vi "AlliGator Fit Linear Combinations of Exponentials.vi"(0 "Fit Simulation Parameters":T13, 5 "Decay Simulation Parameters":T14, 7 "Decay Fit Options & Parameters":T2 {"Fit Options"."Offset Resolution" min=0.0; "Fit Options"."Period" min=0.0; "Fit Options"."Min Decay Percentile" min=0.0 max=1.0; "Fit Options"."Max Decay Percentile" min=0.0 max=100.0; "Fit Parameter Constraints"."Max Value" format="%#.3g"; "Fit Parameter Constraints"."Min Value" format="%#.3g"}, 9 "Reference Decay":cluster{"t Array":dbl[], "IRF Array":dbl[]}, 11 "Error In":errorcluster, 12 "Show Decays, Fits & Residuals":bool) -> (1 "Output Plots":cluster{"t Array":dbl[], "I Array":dbl[]}[](array[cluster]), 2 "Output Plot Names":string[](array[string]), 3 "Plot Colors":u32[](array[colorbox]), 4 "Fit Results":T1[](array[typedef]), 6 "tau 1":dbl[](array[numeric]), 8 "tau 2":dbl[](array[numeric]), 10 "a 1":dbl[](array[numeric]), 14 "Message":string, 15 "Error Out":errorcluster)   [LabVIEW 2021, in "AlliGator Fit Method Benchmark.lvlib"]
doc: "Simulate a 1-Exp or 2-Exp decay and fits it with the selected model."
uses:
  AlliGator Fit Method Benchmark.lvlib
  AlliGator Decay Simulation Parameters.ctl
  AlliGator Fit Simulation Parameters.ctl
  AlliGator Decay Fit Options & Parameters v2.ctl
  Fits/IRF(X)PSED/Decay Fit Options v2.ctl
  Fits/Decay Convolution/Decay Model.ctl
  Fits/Residual Type.ctl
  Fits/IRF(X)PSED/Fit Weights Type.ctl
  Fits/Non-linear Fitting Method v2.ctl
  Fits/Fit Calculation Method.ctl
  Fits/Non-linear Fitting Algorithm.ctl
  AlliGator Decay Fit Parameter Constraints 2.ctl
  Fits/IRF(X)PSED/Decay Fit Parameters In List.ctl
  Fits/IRF(X)PSED/MLE Baseline Offset Type.ctl
  Fits/IRF(X)PSED/IRF(X)PSED Fit Results.ctl
  Histograms/Linear Histogram Options.ctl
  Histograms/Histogram Bin Option.ctl
  Histograms/Histogram Bin Position.ctl
  Graphs/XY Graph/XY Graph Selected Plot Info+Flag.ctl
  Graphs/XY Graph/XY Graph Refnum.ctl
  <vilib>/Utility/miscctls.llb/LVPoint32TypeDef.ctl
  593261b4-01b2-4f61-a03e-748a91d26851.vi
  593261b4-01b2-4f61-a03e-748a91d26851.vi/e021cd17-e000-4244-b7f4-ec50548bdfcb.vi
  593261b4-01b2-4f61-a03e-748a91d26851.vi/b1828c6e-eb0a-43e9-a724-8b596c52e435.vi
  593261b4-01b2-4f61-a03e-748a91d26851.vi/7a6138ed-c001-4311-b538-9ba42ae7c7b1.vi
  593261b4-01b2-4f61-a03e-748a91d26851.vi/52c6b4fa-501b-4af0-803b-8bab516ca5d3.vi
  593261b4-01b2-4f61-a03e-748a91d26851.vi/d7237e10-35ab-4bcb-a0c6-4883c3f4c990.vi
  593261b4-01b2-4f61-a03e-748a91d26851.vi/5fb5dd96-3b97-4592-ba56-58181c8e7105.vi
  593261b4-01b2-4f61-a03e-748a91d26851.vi/8e13a849-a393-4484-9968-4af7b25c38d7.vi
  <vilib>/Utility/error.llb/Error Cluster From Error Code.vi
  AlliGator Abort.vi
  <vilib>/gmath/statdist.llb/Uniform (Discrete) Random.vi
  <userlib>/_OpenG.lib/array/array.llb/Filter 1D Array__ogtk.vi
  <userlib>/_OpenG.lib/array/array.llb/Filter 1D Array (DBL)__ogtk.vi
  <userlib>/_OpenG.lib/array/array.llb/Delete Elements from Array__ogtk.vi
  <userlib>/_OpenG.lib/array/array.llb/Delete Elements from 1D Array (DBL)__ogtk.vi
  <vilib>/ErrorRing/Error Ring.xnode
  Histograms/Histogram Window.lvlib
  Math/Math.lvlib
  GUI/GUI.lvlib
  AlliGator Globals, Variables & Constants.lvlib
  Time/Time.lvlib
  Variant/Variant.lvlib
  AlliGator Decay Fit.lvlib
  Graphs/XY Graph/XY Graph Add-Ons.lvlib
  Fits/Fits.lvlib
  <vilib>/gmath/NI_Gmath.lvlib
  Error/Error.lvlib
  <vilib>/gmath/statdist.llb/Exp Random.vi
  AlliGator Decay Fit Parameter Map.lvlib
panel:
  # "see the AlliGator License on the block diagram (Ctrl+E or Window:Show Block Diagram)"
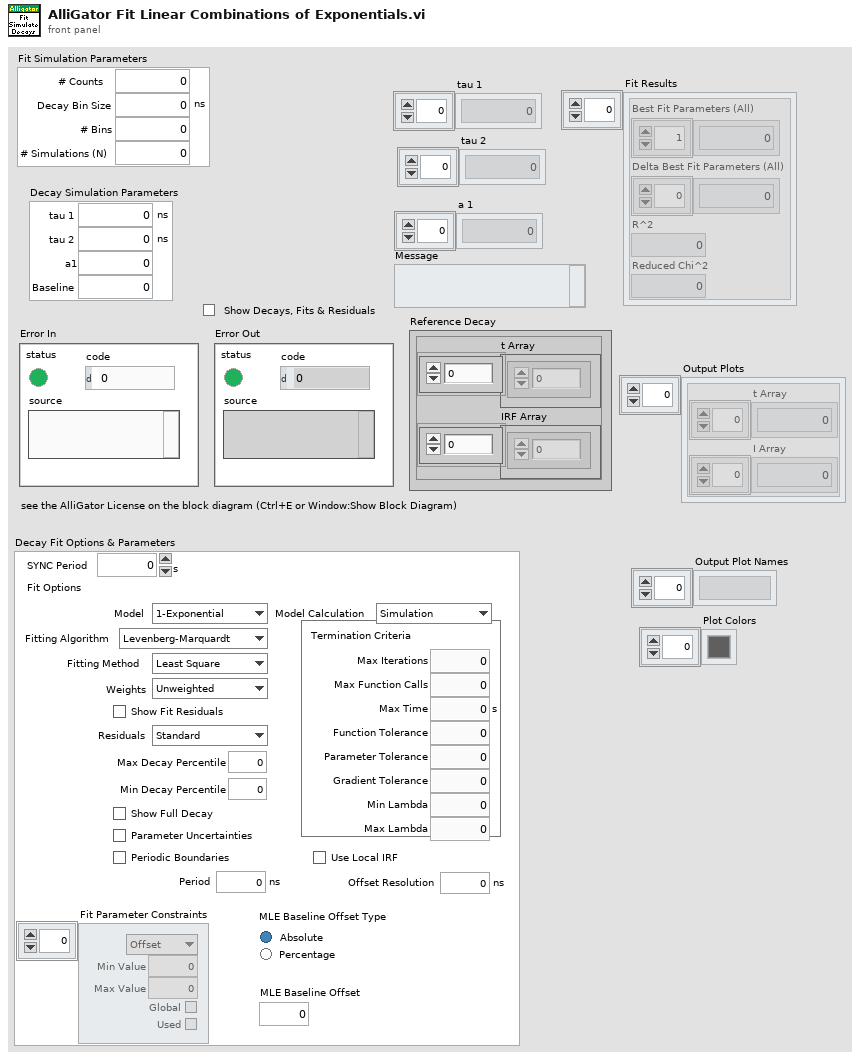
[diagram p1: front panel]
types:
  T1 = typedef "Fits.lvlib/IRF(X)PSED Fit Results.ctl" = cluster{"Best Fit Parameters (All)":dbl[], "Delta Best Fit Parameters (All)":dbl[], "R^2":dbl, "Reduced Chi^2":dbl}
  T2 = typedef "AlliGator Decay Fit Parameter Map.lvlib/AlliGator Decay Fit Options & Parameters v2.ctl" = cluster{"SYNC Period":dbl[unit], "Fit Options":T3, "Fit Parameter Constraints":T10[], "MLE Baseline Offset":dbl, "MLE Baseline Offset Type":T12}
  T3 = typedef "Fits.lvlib/Decay Fit Options v2.ctl" = cluster{"Show Fit Residuals":bool, "Fit Model":T4, "Residual Type":T5, "Max Decay Percentile":dbl, "Min Decay Percentile":dbl, "Show Full Decay":bool, "Weights":T6, "Fitting Method":T7, "Compute Parameter Uncertainties":bool, "Periodic Boundaries":bool, "Model Calculation":T8, "Period":dbl[unit], "Termination Criteria":cluster{"Max Iterations":i32, "Max Function Calls":i32, "Max Time":dbl[unit], "Function Tolerance":dbl, "Parameter Tolerance":dbl, "Gradient Tolerance":dbl, "Min Lambda":dbl, "Max Lambda":dbl, "Initial Tick Count":u32}, "Offset Resolution":dbl[unit], "Use Local IRF":bool, "Fitting Algorithm":T9}
  T4 = typedef "Fits.lvlib/Decay Model.ctl" = enum16{"1-Exponential", "2-Exponentials"}
  T5 = typedef "Fits.lvlib/Residual Type.ctl" = enum16{"Standard", "Normalized", "Reduced"}
  T6 = typedef "Fits.lvlib/Fit Weights Type.ctl" = enum16{"Unweighted", "1/Variance", "Best of All"}
  T7 = typedef "Fits.lvlib/Non-linear Fitting Method v2.ctl" = enum16{"Least Square", "Least Absolute Residual", "Bisquare", "MLE", "-", "Best of All"}
  T8 = typedef "Fits.lvlib/Fit Calculation Method.ctl" = enum16{"Simulation", "Convolution", "Integration"}
  T9 = typedef "Fits.lvlib/Non-linear Fitting Algorithm.ctl" = enum16{"Levenberg-Marquardt", "Trust-Region Dogleg"}
  T10 = typedef "AlliGator Decay Analysis.lvlib/AlliGator Decay Fit.lvlib/AlliGator Decay Fit Parameter Constraints 2.ctl" = cluster{"Fit Parameter":T11, "Min Value":dbl, "Max Value":dbl, "Global":bool, "Used":bool}
  T11 = typedef "Fits.lvlib/Decay Fit Parameters In List.ctl" = enum16{"Offset", "Baseline", "A_1", "tau_1", "A_2", "tau_2"}
  T12 = typedef "Fits.lvlib/MLE Baseline Offset Type.ctl" = enum32{"Absolute", "Percentage"}
  T13 = typedef "AlliGator Fit Method Benchmark.lvlib/AlliGator Fit Simulation Parameters.ctl" = cluster{"# Counts":i32, "# Simulations (N)":i32, "Decay Bin Size":dbl[unit], "# Bins":i32}
  T14 = typedef "AlliGator Fit Method Benchmark.lvlib/AlliGator Decay Simulation Parameters.ctl" = cluster{"tau 1":dbl[unit], "tau 2":dbl[unit], "a1":dbl, "Baseline":dbl}
  T15 = typedef "Histogram Window.lvlib/Linear Histogram Options.ctl" = cluster{"Bin Size":dbl, "Bin Number":i32, "Bin Option":T16, "Min Value":dbl, "Max Value":dbl, "Filter NaN & Infinite Values":bool, "Frequency Plot":bool, "Align Bins":bool, "Bin Location":T17, "Project Outside Values":bool, "Max Histogram Size":i32}
  T16 = typedef "Histogram Window.lvlib/Histogram Bin Option.ctl" = enum32{"Bin Number", "Bin Size"}
  T17 = typedef "Histogram Window.lvlib/Histogram Bin Position.ctl" = enum16{"Left", "Center", "Right"}
  T18 = typedef "XY Graph Add-Ons.lvlib/XY Graph Selected Plot Info+Flag.ctl" = cluster{"Multiplot XY Graph":T19, "Mouse Coordinates":T20, "Plot Index":i32, "Flag":bool}
  T19 = typedef "XY Graph Add-Ons.lvlib/XY Graph Refnum.ctl" = refnum<vi>
  T20 = typedef "LVPoint32TypeDef.ctl" = cluster{"Horizontal":i32, "Vertical":i32}
  T21 = typedef "XY Graph Add-Ons.lvlib/XY Plot Data.ctl" = cluster{"X Array":dbl[], "Y Array":dbl[]}
  T22 = cluster{"t Array":dbl[], "Intensity Array":dbl[]}[]
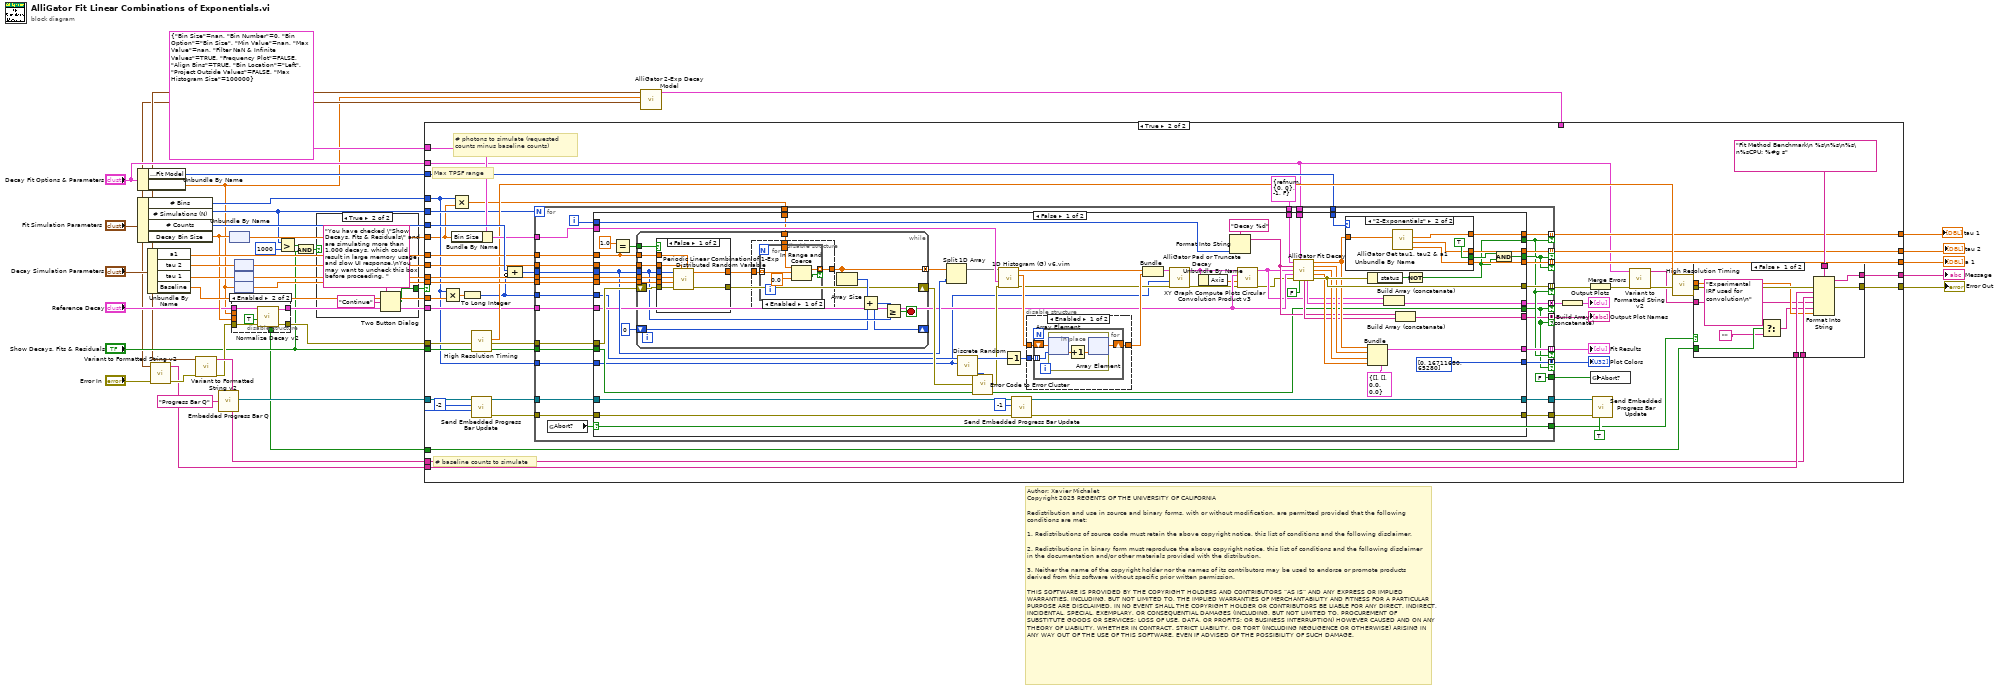
[diagram p0: block diagram]
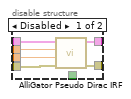
[diagram p2: hidden frame]
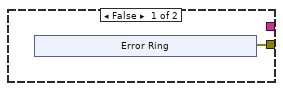
[diagram p3: hidden frame]
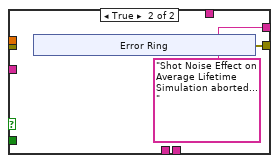
[diagram p4: hidden frame]
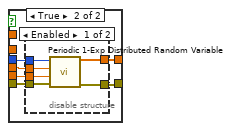
[diagram p6: hidden frame]
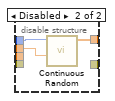
[diagram p7: hidden frame]
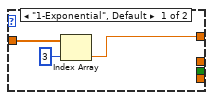
[diagram p9: hidden frame]
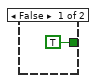
[diagram p11: hidden frame]
diagram:
  # "Author: Xavier Michalet\nCopyright 2025 REGENTS OF THE UNIVERSITY OF CALIFORNIA\n\nRedistribution and use in source and binary forms, with or without modification, are permitted provided that the following conditions are met:\n\n1. Redistributions of source code must retain the above copyright notice, this list of conditions and the following disclaimer.\n\n2. Redistributions in binary form must reproduce the above copyright notice, this list of conditions and the following disclaimer in the documentation and/or other materials provided with the distribution.\n\n3. Neither the name of the copyright holder nor the names of its contributors may be used to endorse or promote products derived from this software without specific prior written permission.\n\nTHIS SOFTWARE IS PROVIDED BY THE COPYRIGHT HOLDERS AND CONTRIBUTORS “AS IS” AND ANY EXPRESS OR IMPLIED WARRANTIES, INCLUDING, BUT NOT LIMITED TO, THE IMPLIED WARRANTIES OF MERCHANTABILITY AND FITNESS FOR A PARTICULAR PURPOSE ARE DISCLAIMED. IN NO EVENT SHALL THE COPYRIGHT HOLDER OR CONTRIBUTORS BE LIABLE FOR ANY DIRECT, INDIRECT, INCIDENTAL, SPECIAL, EXEMPLARY, OR CONSEQUENTIAL DAMAGES (INCLUDING, BUT NOT LIMITED TO, PROCUREMENT OF SUBSTITUTE GOODS OR SERVICES; LOSS OF USE, DATA, OR PROFITS; OR BUSINESS INTERRUPTION) HOWEVER CAUSED AND ON ANY THEORY OF LIABILITY, WHETHER IN CONTRACT, STRICT LIABILITY, OR TORT (INCLUDING NEGLIGENCE OR OTHERWISE) ARISING IN ANY WAY OUT OF THE USE OF THIS SOFTWARE, EVEN IF ADVISED OF THE POSSIBILITY OF SUCH DAMAGE."
  n1 = Unbundle By Name("Decay Fit Options & Parameters") -> ("Fit Options.Fit Model"=w23:T4, "Fit Options.Period"=w2:dbl[unit])
  n2 = Unbundle By Name("Fit Simulation Parameters") -> ("# Bins"=w6:i32, "# Simulations (N)"=w13:i32, "# Counts"=w40:i32, "Decay Bin Size"=w17:dbl[unit])
  n3 = Unbundle By Name("Decay Simulation Parameters") -> ("a1"=w37:dbl, "tau 2"=w35:dbl[unit], "tau 1"=w36:dbl[unit], "Baseline"=w19:dbl)
  n4 = call "Variant to Formatted String v2.vi"("error in (no error)"="Error In", "Anything"="Fit Simulation Parameters") -> ("error out"=w26:errorcluster, "String"=w25:string)  [unwired: 8 in]
  n5 = call "Variant to Formatted String v2.vi"("error in (no error)"=w26, "Anything"="Decay Simulation Parameters") -> ("error out"=w15:errorcluster, "String"=w24:string)  [unwired: 8 in]
  n6 = call "Embedded Progress Bar Q.vi"("Progress Bar Queue Name"="Progress Bar Q") -> ("Progress Bar Queue"=w30:refnum<queue>)  [unwired: 6 in]
  n7 = node(w17) -> (w32:dbl)
  n8 = disable-structure shown="Enabled" {
    disable-tunnel: [w46 w50] -> w18
    disable-tunnel: w17 -> [w45 _]
    disable-tunnel: "Reference Decay" -> [w44 w52]
    disable-tunnel: w15 -> [w43 w51]
    disable-tunnel: [w42 w49] -> w14
    disable-tunnel: w2 -> [w41 _]
    disable-tunnel: [_ w47] -> w5
    frame Disabled {
      n9 = call "AlliGator Pseudo Dirac IRF.vi"("Error In"=w43, "Decay Bin Size"=w45, "Period"=w41, "Reference Decay in"=w44) -> ("Error Out"=w42:errorcluster, "Reference Decay out"=w46:cluster{"t Array":dbl[], "IRF Array":dbl[]})  [unwired: 6 in]
    }
    frame Enabled {
      n10 = call "Normalize Decay v2.vi"("Error In"=w51, "Max = 1 (F)/Integral = 1 (T)"=TRUE, "Decay"=w52) -> ("Error Out"=w49:errorcluster, "Normalized Decay"=w50:cluster{"t Array":dbl[], "Y Array":dbl[]}, "Is Valid Plot?"=w47:bool)  [unwired: 4 in, 2 out]
    }
  }
  n11 = node(w35) -> (w33:dbl)
  n12 = node(w36) -> (w34:dbl)
  n13 = node(w2) -> (w39:dbl)
  n14 = Greater?(x=w13, y=1000) -> (0:w11:bool)
  n15 = And(x=w11, y="Show Decays, Fits & Residuals") -> (x .and. y?=w9:bool)
  n16 = case shown="True" w9 {
    tunnel: [TRUE ("T button?") w54] -> w8
    frame False {
    }
    frame True {
      n17 = Two Button Dialog(message="You have checked \"Show Decays, Fits & Residuals\" and are simulating more than 1,000 decays, which could result in large memory usage and slow UI response.\nYou may want to uncheck this box before proceeding. ", 2:"Continue" ("T button name (\"OK\")")) -> (T button?=w54:bool)  [unwired: 1 in]
    }
  }
  n18 = call "AlliGator 2-Exp Decay Model.vi"("Fit Simulation Parameters"="Fit Simulation Parameters", "Period"=w2, "Decay Simulation Parameters"="Decay Simulation Parameters") -> ("Output Plot"=w1:cluster{"t Array":dbl[], "I Array":dbl[]})  [unwired: 8 in]
  n19 = case shown="True" w8 {
    tunnel: w40 -> [_ w113]
    tunnel: w39 -> [_ w112]
    tunnel: T15 {"Bin Size"=nan, "Bin Number"=0, "Bin Option"=enum."Bin Size", "Min Value"=nan, "Max Value"=nan, "Filter NaN & Infinite Values"=TRUE, "Frequency Plot"=FALSE, "Align Bins"=TRUE, "Bin Location"=enum."Left", "Project Outside Values"=FALSE, "Max Histogram Size"=100000} ("Histogram Options") -> [_ w111]
    tunnel: w37 -> [_ w109]
    tunnel: w34 -> [_ w108]
    tunnel: w33 -> [_ w107]
    tunnel: w32 -> [_ w65]
    tunnel: w30 -> [_ w105]
    tunnel: [w57 w98] -> w29
    tunnel: [_ w97] -> w28
    tunnel: w25 -> [_ w96]
    tunnel: w24 -> [_ w95]
    tunnel: w23 -> [_ w86]
    tunnel: [_ w85] -> w22
    tunnel: [_ w84] -> w21
    tunnel: [_ w83] -> w20
    tunnel: "Decay Fit Options & Parameters" -> [_ w80]
    tunnel: w19 -> [_ w70]
    tunnel: w18 -> [_ w74]
    tunnel: w14 -> [_ w73]
    tunnel: w13 -> [_ w72]
    tunnel: "Show Decays, Fits & Residuals" -> [_ w71]
    tunnel: w6 -> [_ w66]
    tunnel: w5 -> [_ w63]
    tunnel: w1 -> [_ _]
    frame False {
      n20 = xnode "Error Ring"() -> ("error out"=w57:errorcluster)
    }
    frame True {
      # "Max TPSF range"
      # "# photons to simulate (requested counts minus baseline counts)"
      # "# baseline counts to simulate"
      n21 = Multiply(x=w66, y=w70) -> (x*y=w69:dbl)
      n22 = Multiply(x=w66, y=w65) -> (x*y=w64:dbl)
      n23 = Bundle By Name(cluster=w111, "Bin Size"=w65) -> (w110:T15)
      n24 = To Long Integer(number=w69) -> (32bit integer=w67:i32)
      n25 = call "High Resolution Timing.vi"("Error In"=w73) -> ("elapsed (relative) seconds"=w91:dbl, "Error Out"=w93:errorcluster)  [unwired: 16 in, 1 out]
      n26 = call "Send Embedded Progress Bar Update.vi"("Max Iterations N"=w72, "Current Iteration i (i or -1: standard or || iteration; 0 or -2: first standard or || iteration)"=-2 ("Current Iteration i (-1: || iteration, -2: first || iteration)"), "Progress Bar Queue in"=w105) -> ("Error Out"=w102:errorcluster, "Progress Bar Queue out"=w104:refnum<queue>)  [unwired: 7 in]
      n27 = Compound Arithmetic op=ADD(w113, invert w67) -> (w68:i32)
      n28 = for {
        N: w72 -> [_]
        tunnel: w68 -> [w164]
        tunnel: w112 -> [w163]
        tunnel: w93 -> [w162]
        tunnel: w110 -> [w161]
        tunnel: w109 -> [w145]
        tunnel: w108 -> [w160]
        tunnel: w107 -> [w159]
        tunnel: w102 -> [w156]
        tunnel: [w155] -> w101
        tunnel: [FALSE ("Abort?")] -> w99
        tunnel: [w142] -> w89
        tunnel: w74 -> [w153]
        tunnel: w80 -> [w151]
        tunnel: [w144] -> w88 mode=indexing if=w140
        tunnel: T18 {"Multiplot XY Graph"=refnum, "Mouse Coordinates"={"Horizontal"=0, "Vertical"=0}, "Plot Index"=-1, "Flag"=FALSE} ("Selected Plot Info + Flag") -> [w150]
        tunnel: w86 -> [w149]
        tunnel: [w148] -> w85 mode=indexing if=w140
        tunnel: [w147] -> w84 mode=indexing if=w141
        tunnel: [w146] -> w83 mode=indexing if=w141
        tunnel: w104 -> [w158]
        tunnel: [w157] -> w103
        tunnel: [w143] -> w78 mode=indexing if=w140
        tunnel: [w139] -> w76 mode=concatenating if=w132
        tunnel: [w138] -> w77 mode=concatenating if=w132
        tunnel: w71 -> [w137]
        tunnel: [w136] -> w75 mode=concatenating if=w132
        tunnel: w67 -> [w135]
        tunnel: w66 -> [w134]
        tunnel: w64 -> [w133]
        i -> [w152]
        n29 = global read "AlliGator Abort.vi" "Abort?"() -> (w142:bool)
        n30 = case shown="False" w142 {
          tunnel: w164 -> [w177 _]
          tunnel: w163 -> [w227 _]
          tunnel: w162 -> [w226 w294]
          tunnel: w161 -> [w225 _]
          tunnel: w160 -> [w224 _]
          tunnel: w159 -> [w223 _]
          tunnel: w158 -> [w221 w293]
          tunnel: [w220 w293] -> w157
          tunnel: w156 -> [w219 w292]
          tunnel: [w218 w292] -> w155
          tunnel: w153 -> [w175 _]
          tunnel: w152 -> [w217 _]
          tunnel: w151 -> [w215 _]
          tunnel: w150 -> [w213 _]
          tunnel: w149 -> [w212 _]
          tunnel: [w211 _] -> w148
          tunnel: [w210 _] -> w147
          tunnel: [w208 _] -> w146
          tunnel: w145 -> [w207 _]
          tunnel: [w204 w294] -> w144
          tunnel: [w202 _] -> w141
          tunnel: [w201 _] -> w140
          tunnel: [w195 _] -> w143
          tunnel: [w190 _] -> w139
          tunnel: [w191 _] -> w138
          tunnel: [w183 _] -> w132
          tunnel: w137 -> [w183 _]
          tunnel: [u32[] [0, 16711680, 65280] ("Plot Colors (Default)") _] -> w136
          tunnel: w135 -> [w170 _]
          tunnel: w134 -> [w167 _]
          tunnel: w133 -> [w184 _]
          frame False {
            n31 = Equal?(x=1.0, y=w207) -> (x = y?=w206:bool)
            n32 = while {
              tunnel: w227 -> [w242]
              tunnel: w224 -> [w240]
              tunnel: w223 -> [w239]
              tunnel: w207 -> [w238]
              tunnel: w206 -> [w237]
              tunnel: w184 -> [w235]
              tunnel: [w234] -> w182 mode=concatenating
              tunnel: w177 -> [w233]
              shift-right: [w228] -> w179
              shift-left: w226 -> [w241]
              shift-right: [w229] -> _
              shift-left: 0 -> [w230]
              stop <- w232 stop-if-true
              n33 = case shown="False" w237 {
                tunnel: w233 -> [w259 w263]
                tunnel: w242 -> [w258 w261]
                tunnel: w241 -> [w257 w265]
                tunnel: [w256 w260] -> w236
                tunnel: [w255 w264] -> w228
                tunnel: w240 -> [w254 w262]
                tunnel: w239 -> [w253 _]
                tunnel: w238 -> [w252 _]
                frame False {
                  n34 = call "Periodic Linear Combination of 1-Exp Distributed Random Variable.vi"("a 1 (in [0, 1])"=w252, "tau 2"=w253, "Error In"=w257, "T"=w258, "tau 1"=w254, "# Elements"=w259) -> ("Error Out"=w255:errorcluster, "t Array"=w256:dbl[])  [unwired: 4 in]
                }
                frame True {
                  n35 = disable-structure shown="Enabled" {
                    disable-tunnel: w265 -> [w271 _]
                    disable-tunnel: [w270 _] -> w264
                    disable-tunnel: w263 -> [w269 w274]
                    disable-tunnel: w262 -> [w268 w273]
                    disable-tunnel: w261 -> [w267 _]
                    disable-tunnel: [w266 w272] -> w260
                    frame Enabled {
                      n36 = call "Periodic 1-Exp Distributed Random Variable.vi"("Error In"=w271, "T"=w267, "tau"=w268, "# Elements"=w269) -> ("Error Out"=w270:errorcluster, "t Array"=w266:dbl[])  [unwired: 6 in]
                    }
                    frame Disabled {
                      n37 = call-poly <vilib>:"Continuous Random.vi"("b"=w273, "samples"=w274) -> ("exp random data"=w272:dbl[])  [unwired: 8 in, 1 out]
                    }
                  }
                }
              }
              n38 = disable-structure shown="Enabled" {
                disable-tunnel: w236 -> [w245 w251]
                disable-tunnel: w235 -> [w244 _]
                disable-tunnel: [w243 w251] -> w234
                frame Enabled {
                  n39 = for {
                    tunnel: w245 -> [w249] mode=indexing
                    tunnel: w244 -> [w250]
                    tunnel: [w247] -> w243 mode=indexing if=w246
                    n40 = In Range and Coerce(upper limit=w250, x=w249, lower limit=0.0 ("x")) -> (coerced(x)=w247:dbl, In Range?=w246:bool)
                  }
                }
                frame Disabled {
                }
              }
              n41 = Array Size(array=w234) -> (size(s)=w231:i32)
              n42 = Add(x=w231, y=w230) -> (x+y=w229:i32)
              n43 = Greater Or Equal?(x=w229, y=w233) -> (x >= y?=w232:bool)
            }
            n44 = Split 1D Array(array=w182, index=w177) -> (first subarray=w176:dbl[])  [unwired: 1 out]
            n45 = call-poly <vilib>:"Discrete Random.vi"("n"=w167, "samples"=w170) -> ("error"=w180:i32, "uniform (discrete) random data"=w188:i32[])  [unwired: 8 in]
            n46 = call "Error Code to Error Cluster.vi"("Error Code"=w180, "Error In"=w179) -> ("Error Out"=w178:errorcluster)  [unwired: 13 in]
            n47 = call "1D Histogram (G) v6.vim"("Error In"=w178, "Histogram Options"=w225, "Array"=w176) -> ("Error Out"=w169:errorcluster, "Histogram"=w186:dbl[], "Axis"=w171:dbl[])  [unwired: 2 in, 4 out]
            n48 = Decrement(x=w188) -> (x-1=w187:i32[])
            n49 = call "Send Embedded Progress Bar Update.vi"("Error In"=w219, "Current Iteration i (i or -1: standard or || iteration; 0 or -2: first standard or || iteration)"=-1 ("Current Iteration i (i or -1: standard or || iteration; 0 or -2: first standard or || iteration)"), "Progress Bar Queue in"=w221) -> ("Error Out"=w218:errorcluster, "Progress Bar Queue out"=w220:refnum<queue>)  [unwired: 7 in]
            n50 = disable-structure shown="Enabled" {
              disable-tunnel: w187 -> [w277 _]
              disable-tunnel: w186 -> [w276 w283]
              disable-tunnel: [w275 w283] -> w185
              frame Enabled {
                n51 = for {
                  tunnel: w277 -> [w278] mode=indexing
                  shift-right: [w279] -> w275
                  shift-left: w276 -> [w280]
                  n52 = in-place {
                    n53 = in-place-array #1(w280, w278) -> (w282:dbl)
                    n54 = Increment(x=w282) -> (x+1=w281:dbl)
                    n55 = in-place-array #1(w281) -> (w279:dbl[])  [unwired: 1 out]
                  }
                }
              }
              frame Disabled {
              }
            }
            n56 = Bundle("Axis"=w171, "Histogram"=w185) -> (w172:cluster{"Axis":dbl[], "Histogram":dbl[]})  [unwired: 1 in]
            n57 = call "AlliGator Pad or Truncate Decay.vi"("Error In"=w169, "# Requested Points"=w167, "Plot in"=w172) -> ("Error Out"=w168:errorcluster, "Plot out"=w166:cluster{"Axis":dbl[], "Histogram":dbl[]})  [unwired: 7 in]
            n58 = Unbundle By Name(w166) -> ("Axis"=w165:dbl[])
            n59 = Format Into String(format string="Decay %d", w217) -> (resulting string=w189:string)  [unwired: 2 in, 1 out]
            n60 = call "XY Graph Compute Plots Circular Convolution Product v3.vi"("Error In"=w168, "Support Axis (kernel's)"=w165, "Plot 2 (kernel)"=w175, "Plot 1 (function)"=w166) -> ("Error Out"=w173:errorcluster, "Convolution Product"=w174:T21)  [unwired: 5 in, 1 out]
            n61 = call "AlliGator Fit Decay.vi"("Selected Plot Info + Flag"=w213, "Decay Fit Options & Parameters"=w215, "Current Decay Name"=w189, "Current Decay"=w174, "Reference Decay"=w175, "error in (no error)"=w173, "Use Legacy Fitting Approach"=FALSE) -> ("Output Plots"=w193:T22, "Best Fit Parameters (All)"=w200:dbl[], "Delta Best Fit Parameters (All)"=w199:dbl[], "R^2"=w198:dbl, "Reduced Chi^2"=w197:dbl, "Output Plot Names"=w194:string[], "Error Out"=w204:errorcluster)  [unwired: 2 out]
            n62 = case shown="\"2-Exponentials\"" w212 {
              tunnel: w200 -> [w286 w290]
              tunnel: [w284 w289] -> w211
              tunnel: [_ w288] -> w210
              tunnel: [_ TRUE] -> w209
              tunnel: [_ w287] -> w208
              frame "1-Exponential", Default {
                n63 = Index Array(array=w286, index=3) -> (element=w284:dbl)
              }
              frame "2-Exponentials" {
                n64 = call "AlliGator Get tau1, tau2 & a1.vi"("Best Fit Parameters"=w290) -> ("a 1"=w287:dbl, "tau 2"=w288:dbl, "tau 1"=w289:dbl)  [unwired: 8 in]
              }
            }
            n65 = Unbundle By Name(w204) -> ("status"=w203:bool)
            n66 = Bundle(cluster=T1 {"Best Fit Parameters (All)"=[], "Delta Best Fit Parameters (All)"=[], "R^2"=0.0, "Reduced Chi^2"=0.0} ("output cluster"), "Best Fit Parameters (All)"=w200, "Delta Best Fit Parameters (All)"=w199, "R^2"=w198, "Reduced Chi^2"=w197) -> (w195:T1)
            n67 = Build Array (concatenate)(w174, w193) -> (w191:T21[])
            n68 = Build Array (concatenate)(w189, w194) -> (w190:string[])
            n69 = Not(x=w203) -> (.not. x?=w201:bool)
            n70 = And(x=w209, y=w201) -> (x .and. y?=w202:bool)
          }
          frame True {
          }
        }
      }
      "Fit Results" <- w78
      "Output Plot Names" <- w76
      "Plot Colors" <- w75
      n71 = Build Array (concatenate)(w77) -> (→"Output Plots":T21[])
      n72 = Merge Errors(w88) -> (w82:errorcluster)
      n73 = global write "AlliGator Abort.vi" "Abort?"(w99) -> ()
      n74 = call "Send Embedded Progress Bar Update.vi"("Stop Progress Bar (F)"=TRUE, "Error In"=w101, "Progress Bar Queue in"=w103) -> ()  [unwired: 7 in, 2 out]
      n75 = call "Variant to Formatted String v2.vi"("error in (no error)"=w82, "Anything"=w80) -> ("error out"=w81:errorcluster, "String"=w79:string)  [unwired: 8 in]
      n76 = call "High Resolution Timing.vi"("relative seconds (NaN)"=w91, "Error In"=w81) -> ("elapsed (relative) seconds"=w90:dbl, "Error Out"=w92:errorcluster)  [unwired: 15 in, 1 out]
      n77 = case shown="False" w89 {
        tunnel: [w125 w126] -> w98
        tunnel: [w124 "Shot Noise Effect on Average Lifetime Simulation aborted..."] -> w97
        tunnel: w96 -> [w123 _]
        tunnel: w95 -> [w122 _]
        tunnel: "Fit Method Benchmark\n %s\n%s\n%s\n%sCPU: %#g s" ("format string") -> [w121 _]
        tunnel: w92 -> [w120 _]
        tunnel: w90 -> [w119 _]
        tunnel: w79 -> [w118 _]
        tunnel: w63 -> [w117 _]
        frame False {
          n78 = Select(t="Experimental IRF used for convolution\n", s=w117, f="") -> (s? t:f=w116:string)
          n79 = Format Into String(format string=w121, error in=w120, w123, w122, w118, w116, w119) -> (resulting string=w124:string, error out=w125:errorcluster)  [unwired: 1 in]
        }
        frame True {
          n80 = xnode "Error Ring"() -> ("error out"=w126:errorcluster)
        }
      }
    }
  }
  "Error Out" <- w29
  "a 1" <- w20
  "tau 1" <- w22
  "tau 2" <- w21
  "Message" <- w28
